vi "DAQ Output.vi"(10 "Numeric":dbl format="%#_13g") -> ()   [LabVIEW 2018]
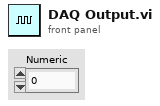
[diagram p1: front panel]
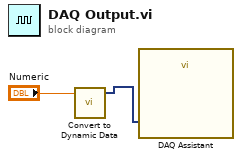
[diagram p0: block diagram]
diagram:
  n1 = call "Convert to Dynamic Data"("Double"="Numeric") -> ("Dynamic Data Type"=w1:dynamicdata)  [unwired: 3 in]
  n2 = call "DAQ Assistant"("data"=w1) -> ()  [unwired: 17 in, 2 out]
